vi "Write HGF_Configuration.vi"(8 "error in (no error)":errorcluster, 10 "HGF_Configuration":refnum<class "HGF_Configuration.lvclass">, 11 "HGF_Application in":refnum<class "HGF_Application.lvclass">) -> (0 "error out":errorcluster, 3 "HGF_Application out":refnum<class "HGF_Application.lvclass">)   [LabVIEW 2012, in "HGF_ApplicationBaseClasses.lvlib" / "HGF_Application.lvclass"]
uses:
  HGF_Application.lvclass
  HGF_Configuration/HGF_Configuration.lvclass
  HGF_Application.lvclass/HGF_Application.ctl
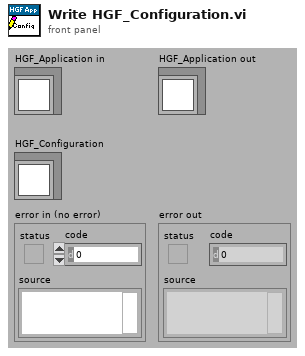
[diagram p1: front panel]
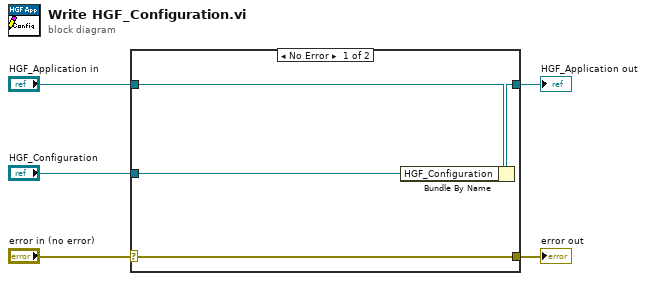
[diagram p0: block diagram]
diagram:
  n1 = case shown="No Error" "error in (no error)" {
    selector: "error in (no error)" -> [w9 w10]
    tunnel: [w9 w10] -> w4
    tunnel: [w7 w11] -> w2
    tunnel: "HGF_Application in" -> [w8 w11]
    tunnel: "HGF_Configuration" -> [w6 _]
    frame No Error {
      n2 = Bundle By Name(cluster=w8, "HGF_Configuration"=w6) -> (w7:refnum<class "HGF_Application.lvclass">)
    }
    frame Error {
    }
  }
  "error out" <- w4
  "HGF_Application out" <- w2
